vi "Set Scaling Factor.vi"(8 "error in (no error)":errorcluster, 10 "Value":dbl, 11 "QRCodeDetector in":refnum<class "QRDetector.lvclass">) -> (0 "error out":errorcluster, 3 "QRCodeDetector (Duplicate)":refnum<class "QRDetector.lvclass">)   [LabVIEW 2020, in "g_ar_toolkit.feature_detection.lvlib" / "QRDetector.lvclass"]
uses:
  QRDetector.lvclass
  QRDetector.lvclass/QRDetector.ctl
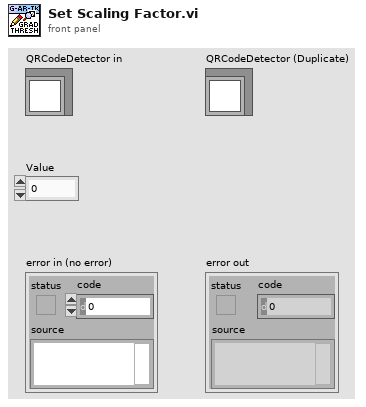
[diagram p1: front panel]
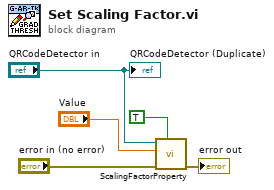
[diagram p0: block diagram]
diagram:
  n1 = call "ScalingFactorProperty.vi"("Write?"=TRUE, "error in (no error)"="error in (no error)", "Value in"="Value", "QRCodeDetector in"="QRCodeDetector in") -> ("error out"=→"error out":errorcluster)  [unwired: 6 in, 1 out]
  "QRCodeDetector (Duplicate)" <- "QRCodeDetector in"
